vi "gDetector.vi"() -> ()   [LabVIEW 2024]
uses:
  Type Definitions.llb/ListOfDetectors.ctt
panel:
  in  "FPN Filter":bool
  in  "PDA Accumulations":i32=1 min=1
  in  "PDA OK?":bool
  out "Current Detector":T1
  in  "CCD OK?":bool
  in  "CCD Setup String":string="LDu,0,256,8;SDu,0,1024,1024;CL4;OMrm;SRon"
  # "Detector Controls"
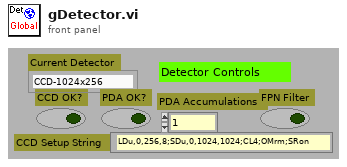
[diagram p1: front panel]
types:
  T1 = typedef "ListOfDetectors.ctt" = enum8{"CCD-1024x256", "InGaAs PDA-1024x1", "CCD-1340x400", "Ge Single Channel", "Si Single Channel", "PMT Single Channel"}
diagram:
